vi "Write Footer To Log File.vi"(5 "Module Close Timestamp":timestamp, 7 "Module Init Timestamp":timestamp, 8 "Error In":errorcluster, 9 "Total no. of errors handled":i32, 10 "Total no. of errors reported":i32, 11 "Error_Log_Setting":T1) -> (0 "Error Out":errorcluster)   [LabVIEW 2023, in "Error Manager.lvlib" / "Error Log.lvclass"]
doc: "This VI logs (writes) a footer message to the Error Log file.\n\nThe footer message is the last message that the Error Manager writes to the log file. The footer is written just before the log file reference is closed."
uses:
  Error Log.lvclass
  Settings/Error_Log_Setting (enum).ctl
  Settings/Settings.lvclass
panel:
  out "Number of characters":i32
  out "Text written to log":string
  # "Input\nInputs to the VI"
  # "Development\nControls or indicators that are useful for development or testing, but which are not outputs of the VI."
  # "Output\nOutputs of the VI"
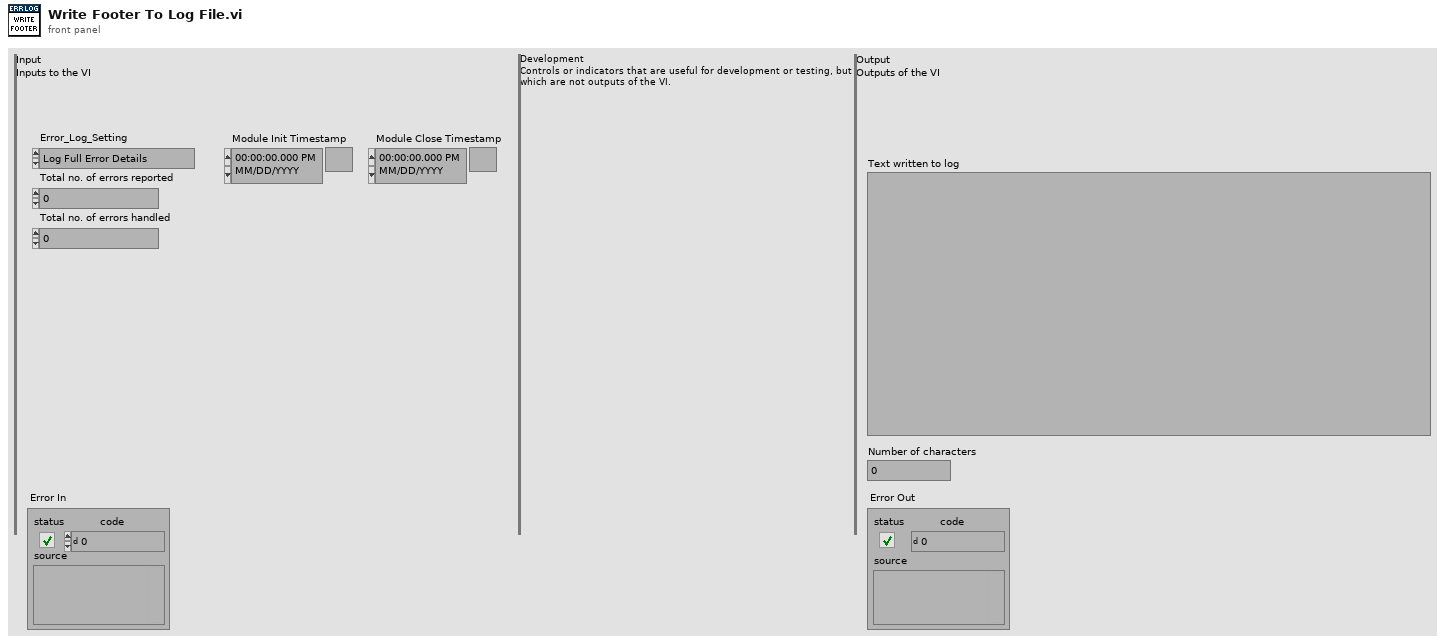
[diagram p1: front panel]
types:
  T1 = typedef "Error Manager.lvlib/Settings.lvclass/Error_Log_Setting (enum).ctl" = enum16{"Log Full Error Details", "Log Error Codes Only", "Do Not Log"}
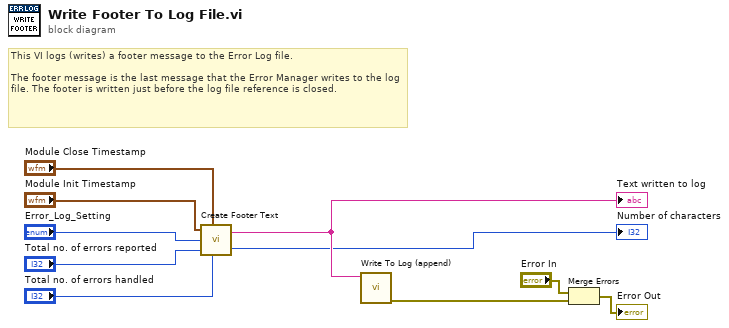
[diagram p0: block diagram]
diagram:
  # "This VI logs (writes) a footer message to the Error Log file.\n\nThe footer message is the last message that the Error Manager writes to the log file. The footer is written just before the log file reference is closed."
  n1 = call "Create Footer Text.vi"("Module Init Timestamp"="Module Init Timestamp", "Module Close Timestamp"="Module Close Timestamp", "Error_Log_Setting"="Error_Log_Setting", "Total no. of errors reported"="Total no. of errors reported", "Total no. of errors handled"="Total no. of errors handled") -> ("Footer to be written to error log file"=w7:string, "Number of characters"=→"Number of characters":i32)
  "Text written to log" <- w7
  n2 = call "Write To Log (append).vi"("Text to write"=w7) -> ("error out"=w8:errorcluster)  [unwired: 10 in]
  n3 = Merge Errors("Error In", w8) -> (→"Error Out":errorcluster)
